vi "set_shutter.vi"(8 "error in (no error)":errorcluster, 10 "shutter open?":bool=TRUE, 11 "LightSourceAN191011Chameleon in":refnum<class "LightSourceAN191011Chameleon.lvclass">) -> (0 "error out":errorcluster, 2 "shutter status":bool, 3 "LightSourceAN191011Chameleon out":refnum<class "LightSourceAN191011Chameleon.lvclass">)   [LabVIEW 2010, in "LightSourceAN191011Chameleon.lvclass"]
uses:
  LightSourceAN191011Chameleon.lvclass
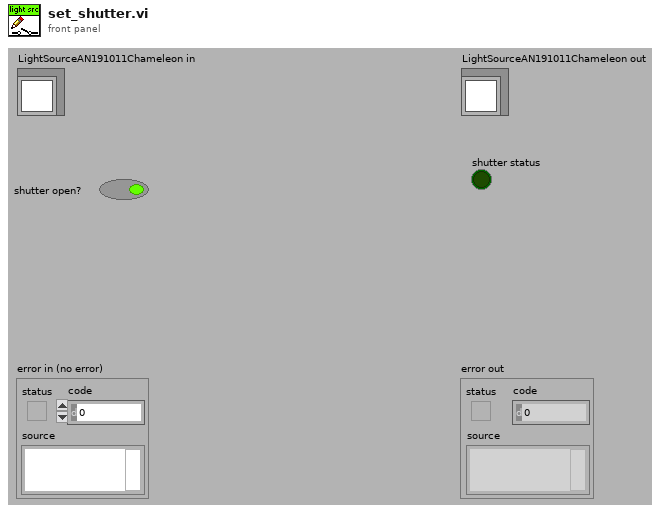
[diagram p1: front panel]
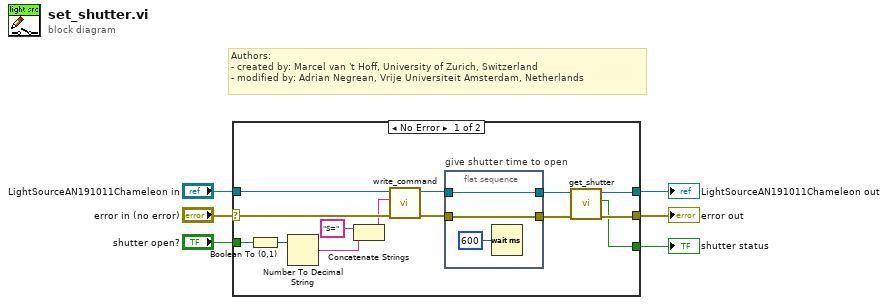
[diagram p0: block diagram]
diagram:
  # "Authors: \n- created by: Marcel van 't Hoff, University of Zurich, Switzerland\n- modified by: Adrian Negrean, Vrije Universiteit Amsterdam, Netherlands"
  n1 = case shown="No Error" "error in (no error)" {
    selector: "error in (no error)" -> [w20 w25]
    tunnel: [w8 w25] -> w5
    tunnel: [w9 w24] -> w2
    tunnel: "LightSourceAN191011Chameleon in" -> [w19 w24]
    tunnel: "shutter open?" -> [w17 _]
    tunnel: [w7 _] -> w1
    frame No Error {
      n2 = Boolean To (0,1)(Boolean=w17) -> (0, 1=w18:i16)
      n3 = Number To Decimal String(number=w18) -> (decimal integer string=w15:string)  [unwired: 1 in]
      n4 = Concatenate Strings("S=" ("string"), w15) -> (w14:string)
      n5 = call-dynamic "write_command.vi"("error in (no error)"=w20, "string to write"=w14, "LightSourceAN191011Chameleon in"=w19) -> ("error out"=w12:errorcluster, "LightSourceAN191011Chameleon out"=w13:refnum<class "LightSourceAN191011Chameleon.lvclass">)  [unwired: 6 in, 1 out]
      n6 = flat-sequence "give shutter time to open" {
        tunnel: w13 -> [w22]
        tunnel: w12 -> [w23]
        tunnel: [w23] -> w10
        tunnel: [w22] -> w11
        frame #0 {
          n7 = Wait (ms)(milliseconds to wait=u32 600) -> ()  [unwired: 1 out]
        }
      }
      n8 = call-dynamic "get_shutter.vi"("error in (no error)"=w10, "LightSourceAN191011Chameleon in"=w11) -> ("error out"=w8:errorcluster, "shutter status"=w7:bool, "LightSourceAN191011Chameleon out"=w9:refnum<class "LightSourceAN191011Chameleon.lvclass">)  [unwired: 7 in]
    }
    frame Error {
    }
  }
  "error out" <- w5
  "LightSourceAN191011Chameleon out" <- w2
  "shutter status" <- w1
